vi "CoordSystem_Convert_Translation3d.vi"(9 "CoordSys To":T1={"Rotation"={"Q_quaternion"={"R"=1.0, "V"=[0.0, 0.0, 0.0]}}}, 10 "CoordSys From":T1={"Rotation"={"Q_quaternion"={"R"=1.0, "V"=[0.0, 0.0, 0.0]}}}, 11 "in Translation3d":T4 {"Z" format="%14.3f"; "Y" format="%14.3f"; "X" format="%14.3f"}) -> (3 "out Converted Translation3d":T4 {"Z" format="%14.3f"; "Y" format="%14.3f"; "X" format="%14.3f"})   [LabVIEW 2019, in "Trajectory_Library.lvlib"]
doc: "Converts the given translation from one coordinate system to another.\n\nInputs:\n - in translation3d -- The translation to convert.\n - Coord Sys from -- The coordinate system the pose starts in.\n - Coord Sys to -- The coordinate system to which to convert.\n\nReturns:\n - Converted Translation -- The given translation in the desired coordinate system."
uses:
  Trajectory_Library.lvlib
  TRANSLATION3D.ctl
  COORDINATE_SYSTEM.ctl
  ROTATION3D.ctl
  QUATERNION.ctl
  Rotation3d_UnaryMinus.vi
  Rotation3d_RotateBy.vi
  Rotation3d_GetQuaterion.vi
  Quaternion_New.vi
  Quaternion_Times.vi
  Quaternion_Inverse.vi
  Quaternion_Get_All.vi
  Rotation3d_Create_Quaternion.vi
  Quaternion_Normalize.vi
  Quaternion_New_Default.vi
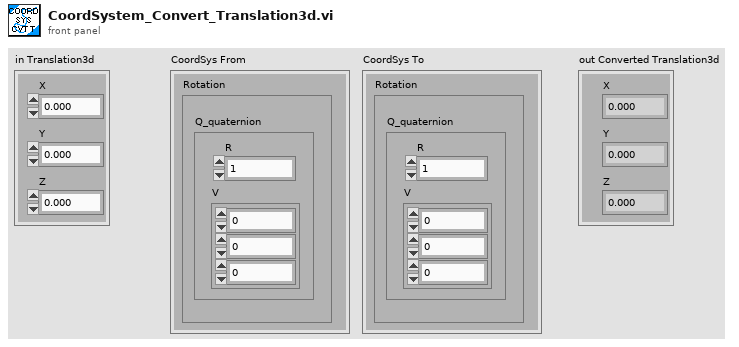
[diagram p1: front panel]
types:
  T1 = typedef "Trajectory_Library.lvlib/COORDINATE_SYSTEM.ctl" = cluster{"Rotation":T2}
  T2 = typedef "Trajectory_Library.lvlib/ROTATION3D.ctl" = cluster{"Q_quaternion":T3}
  T3 = typedef "Trajectory_Library.lvlib/QUATERNION.ctl" = cluster{"R":dbl, "V":dbl[]}
  T4 = typedef "Trajectory_Library.lvlib/TRANSLATION3D.ctl" = cluster{"X":dbl, "Y":dbl, "Z":dbl}
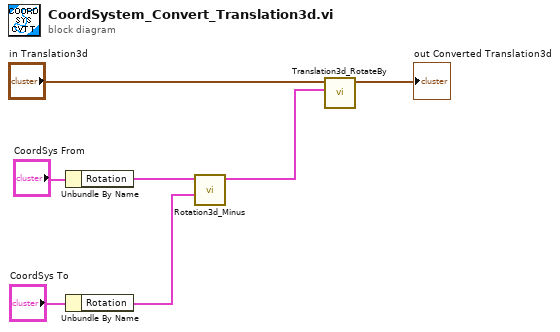
[diagram p0: block diagram]
diagram:
  n1 = Unbundle By Name("CoordSys From") -> ("Rotation"=w3:T2)
  n2 = Unbundle By Name("CoordSys To") -> ("Rotation"=w2:T2)
  n3 = call "Rotation3d_Minus.vi"("other Rotation3d"=w2, "in Rotation3d"=w3) -> ("out Rotation3d"=w1:T2)  [unwired: 9 in]
  n4 = call "Translation3d_RotateBy.vi"("other Rot3d"=w1, "in Translation3D"="in Translation3d") -> ("out Translation3d"=→"out Converted Translation3d":T4)  [unwired: 9 in]
